vi "Test Process Async Request.vi"(8 "error in (no error)":errorcluster, 11 "Process Test In":refnum<class "Process Dev Test.lvclass">) -> (0 "error out":errorcluster, 3 "Process Test Out":refnum<class "Process Dev Test.lvclass">)   [LabVIEW 2020, in "Process Dev Test.lvclass"]
uses:
  Process Dev Test.lvclass
  C:/Program Files (x86)/National Instruments/LabVIEW 2020/vi.lib/Astemes/LUnit/Test Case.lvclass
  source/Framework Test Suite/Mock Process/Mock Process.lvclass
  C:/git/astemes-triarc-framework/source/Framework/Process/Process.lvclass
  source/Framework/Synchronous Request Callback/Synchronous Request Callback.lvclass/Synchronous Request Callback.ctl
  <vilib>/Astemes/LUnit/Test Case.lvclass/Test Case.ctl
  source/Framework/Process/Process.lvclass/Process.ctl
  524619f8-7473-454a-a6a7-9ecc70236b1e.vi
  <vilib>/Astemes/LUnit/Append Pass Result.vi
  <vilib>/Astemes/LUnit/Append Fail Result.vi
  <vilib>/Astemes/LUnit/Describe Comparison.vi
  <vilib>/Astemes/LUnit/Compare Variants.vi
  source/Framework/Process/Private/SubVIs/Wait for finish.vi
  source/Framework/Process/Private/SubVIs/Set Lifecycle State.vi
  source/Framework/Process/Protected/Messaging/Send Message.vi
  source/Framework/Process/Public/Lifecycle/Get Lifecycle State.vi
  <vilib>/Astemes/LUnit/Variant to string.vi
  source/Framework/Process/Private/SubVIs/Handle Debug Data.vi
  <vilib>/Utility/error.llb/Clear Errors.vi
  source/Framework/Logging/Log Debug.vi
  <vilib>/AdvancedString/1D String Array to Delimited String.vi
  <vilib>/Utility/High Resolution Relative Seconds.vi
  source/Framework/Synchronous Request Callback/Synchronous Request Callback.lvclass
  C:/git/astemes-triarc-framework/source/Framework/Callback/Callback.lvclass
  <vilib>/Utility/Data Type/Get Type Information.vi
  <vilib>/Utility/LVClass/Get LV Class Name.vi
  <vilib>/Utility/error.llb/Error Cluster From Error Code.vi
  source/Framework/Process/Public/Read Name.vi
  source/Framework/Callback/Callback.lvclass
  source/Framework/Process/Process.lvclass
  Process Dev Test.lvclass/Process Dev Test.ctl
  C:/git/astemes-triarc-framework/source/Framework/Base/Base.lvclass
  C:/git/astemes-triarc-framework/source/Framework/Configuration File/Configuration File.lvclass
  C:/git/astemes-triarc-framework/source/Framework/Configuration/Configuration.lvclass
  C:/git/astemes-triarc-framework/source/Framework/Error Handler Interface/Error Handler Interface.lvclass
  C:/git/astemes-triarc-framework/source/Framework/Logging/Logging.lvclass
  C:/git/astemes-triarc-framework/source/Framework Test Suite/Mock Process/Mock Process.lvclass
  C:/git/astemes-triarc-framework/source/Framework/Async Handler/Async Handler.lvclass
  C:/git/astemes-triarc-framework/source/Framework/Helper Loop/Helper Loop.lvclass
  C:/git/astemes-triarc-framework/source/Framework/Synchronous Request Callback/Synchronous Request Callback.lvclass
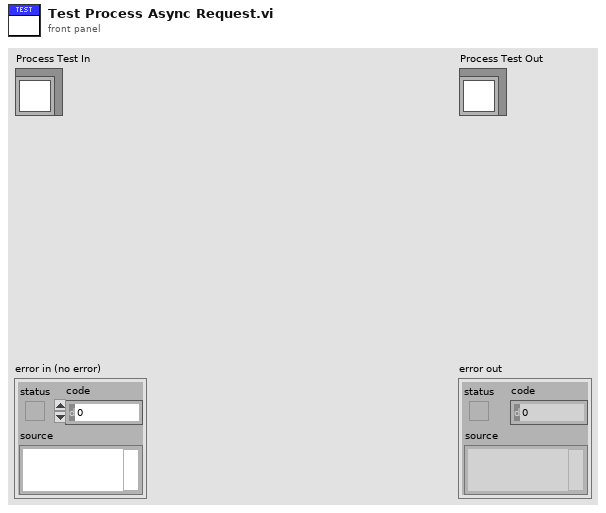
[diagram p1: front panel]
types:
  T1 = cluster{"Request Message":string, "Request Message Data":variant}
  T2 = typedef "Synchronous Request Callback.lvclass/Response Message Cluster.ctl" = cluster{"Message":string, "Message Data":variant, "Error Out":errorcluster}
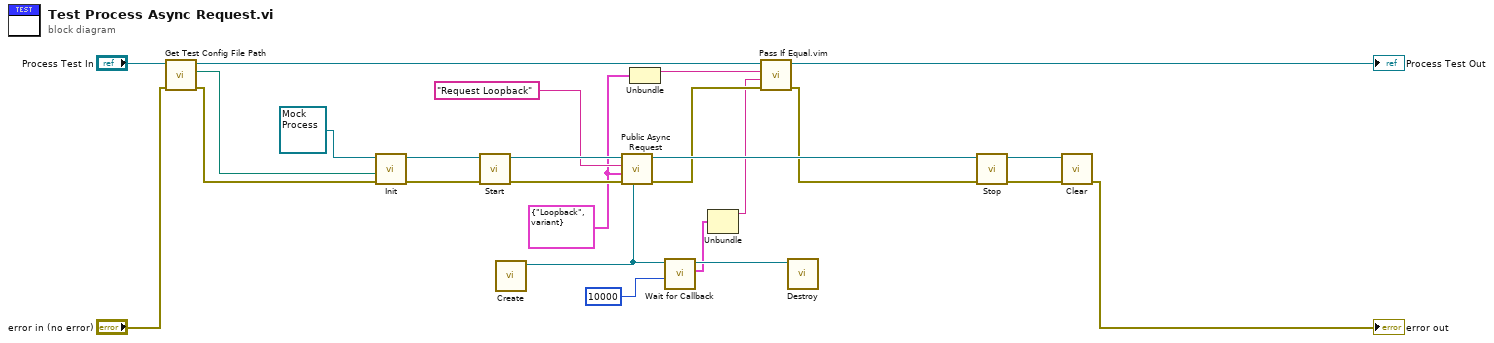
[diagram p0: block diagram]
diagram:
  w2 = T1 {"Request Message"="Loopback", "Request Message Data"=variant} ("output cluster")
  n1 = call "Get Test Config File Path.vi"("error in (no error)"="error in (no error)", "Process Test In"="Process Test In") -> ("error out"=w19:errorcluster, "Test config path"=w20:path, "Process Test Out"=w12:refnum<class "Process Dev Test.lvclass">)  [unwired: 7 in]
  n2 = call-dynamic "Init.vi"("error in (no error)"=w19, "Config File Path"=w20, "Mock Process In"=refnum<class "Mock Process.lvclass"> refnum ("Mock Process.lvclass")) -> ("error out"=w22:errorcluster, "Mock Process Out"=w23:refnum<class "Mock Process.lvclass">)  [unwired: 7 in]
  n3 = call "Start.vi"("error in (no error)"=w22, "Process In"=w23) -> ("error out"=w16:errorcluster, "Process Out"=w14:refnum<class "Mock Process.lvclass">)  [unwired: 7 in, 1 out]
  n4 = call "Create.vi"() -> ("Synchronous Request Callback Out"=w7:refnum<class "Synchronous Request Callback.lvclass">)  [unwired: 10 in, 1 out]
  n5 = call "Public Async Request.vi"("Callback"=w7, "error in (no error)"=w16, "Request Message Data"=w2, "Request Message"="Request Loopback", "Mock Process In"=w14) -> ("error out"=w10:errorcluster, "Mock Process Out"=w13:refnum<class "Mock Process.lvclass">)  [unwired: 5 in]
  n6 = Unbundle(w2) -> ("Request Message"=w1:string)  [unwired: 1 out]
  n7 = call "Wait for Callback.vi"("timeout in ms (-1)"=10000, "Synchronous Request Callback In"=w7) -> ("notification"=w5:T2, "Synchronous Request Callback Out"=w6:refnum<class "Synchronous Request Callback.lvclass">)  [unwired: 6 in, 2 out]
  n8 = Unbundle(w5) -> ("Message"=w4:string)  [unwired: 2 out]
  n9 = call "Pass If Equal.vim"("error in (no error)"=w10, "Actual"=w4, "Expected"=w1, "LUnit Test Case In"=w12) -> ("error out"=w8:errorcluster, "LUnit Test Case Out"=→"Process Test Out":refnum<class "Process Dev Test.lvclass">)  [unwired: 6 in]
  n10 = call "Destroy.vi"("Synchronous Request Callback In"=w6) -> ()  [unwired: 10 in, 1 out]
  n11 = call "Stop.vi"("error in (no error)"=w8, "Process In"=w13) -> ("error out"=w15:errorcluster, "Process Out"=w25:refnum<class "Mock Process.lvclass">)  [unwired: 7 in, 1 out]
  n12 = call-dynamic "Clear.vi"("error in (no error)"=w15, "Mock Process In"=w25) -> ("error out"=→"error out":errorcluster)  [unwired: 9 in]
